vi "get_package_attribute_string.vi"(8 "error in (no error)":errorcluster, 10 "package_manager":string="nipm", 11 "dragon_file_path":path=path "C:/Projects/labview-project-load-tools/rust_src/toml_edit_dll/lv_src/test.toml") -> ()   [LabVIEW 2020]
uses:
  dragon_toml_32.dll
panel:
  in  "attribute_name":string="version"
  in  "package_name":string="ni-daqmx"
  out "value":string
  out "error out":errorcluster
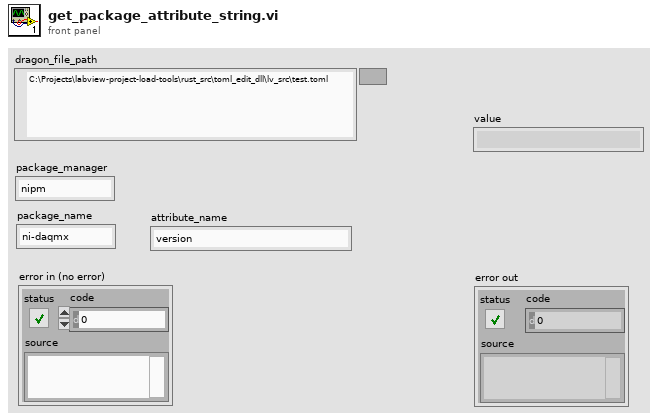
[diagram p1: front panel]
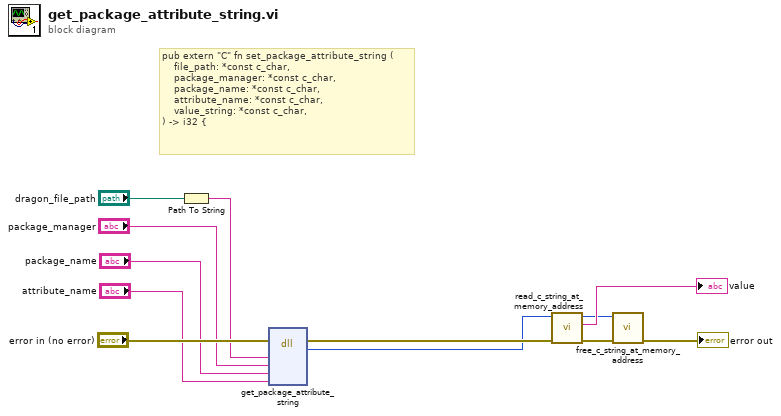
[diagram p0: block diagram]
diagram:
  # "pub extern \"C\" fn set_package_attribute_string (\n    file_path: *const c_char,\n    package_manager: *const c_char,\n    package_name: *const c_char,\n    attribute_name: *const c_char,\n    value_string: *const c_char,\n) -> i32 {"
  n1 = Path To String(path="dragon_file_path") -> (string=w9:string)
  n2 = dll-call lib="C:/Projects/labview-project-load-tools/rust_src/toml_edit_dll/lv_src/dragon_toml_*.dll" fn="get_package_attribute_string"(error in="error in (no error)", "file_path"=w9, "package_manager"="package_manager", "package_name"="package_name", "attribute_name"="attribute_name") -> (error out=w7:errorcluster, "result"=w4:u64)  [unwired: 6 in, 1 out]
  n3 = call "read_c_string_at_memory_address.vi"("error in (no error)"=w7, "memory_address"=w4) -> ("error out"=w8:errorcluster, "string"=→"value":string, "memory_address out"=w3:u64)  [unwired: 7 in]
  n4 = call "free_c_string_at_memory_address.vi"("error in (no error)"=w8, "memory_address"=w3) -> ("error out"=→"error out":errorcluster)  [unwired: 9 in]
